vi "ziPollData.vi"(8 "Error In":errorcluster, 9 "Data In":T1, 10 "TimeOut ms (50)":i32=50, 11 "Handle In":T3 {"Handle" format="0x%08x"; "Conn" format="0x%08x"}) -> (0 "Error Out":errorcluster, 1 "Data Out":T1, 2 "PathArray":string[](array[string]), 3 "Handle Out":T3 {"Handle" format="0x%08x"; "Conn" format="0x%08x"}, 5 "Timed Out":bool, 7 "ziDataType":T4)   [LabVIEW 2015, in "Zurich Instruments LabOne.lvlib"]
doc: "This vi is <b>obsolete</b>. Use ziPollDataEx.vi in combination with ziGetEvent.vi instead.\n\nThis vi returns immediately if data is pending. Otherwise it waits for data for up to <b>TimeOut</b> milliseconds. All value changes that occur in nodes that have been subscribed to or in children of nodes that have been subscribed to, are sent from the Data Server to the ziAPI session. When no event was available within <b>TimeOut</b> milliseconds, the ziValueType field will be ZI_DATA_NONE and <b>Timed Out</b> will be true. Otherwise these fields hold the values corresponding to the event occurred."
uses:
  Zurich Instruments LabOne.lvlib
  Zurich Instruments/LabOne/API/LabVIEW/Zurich Instruments LabOne/Private/ziLV64.framework
  ziGetEventAuxInSample.vi
  ziGetEventDIOSample.vi
  ziGetEventScopeWave.vi
  ziGetEventByteArray.vi
  ziGetEventTreeChange.vi
  ziTypeDemodSample.ctl
  ziTypeHandle.ctl
  ziTypePollData.ctl
  ziTypePollType.ctl
panel:
  # "Obsolete (2013-11)\nUse ziPollDataEx instead"
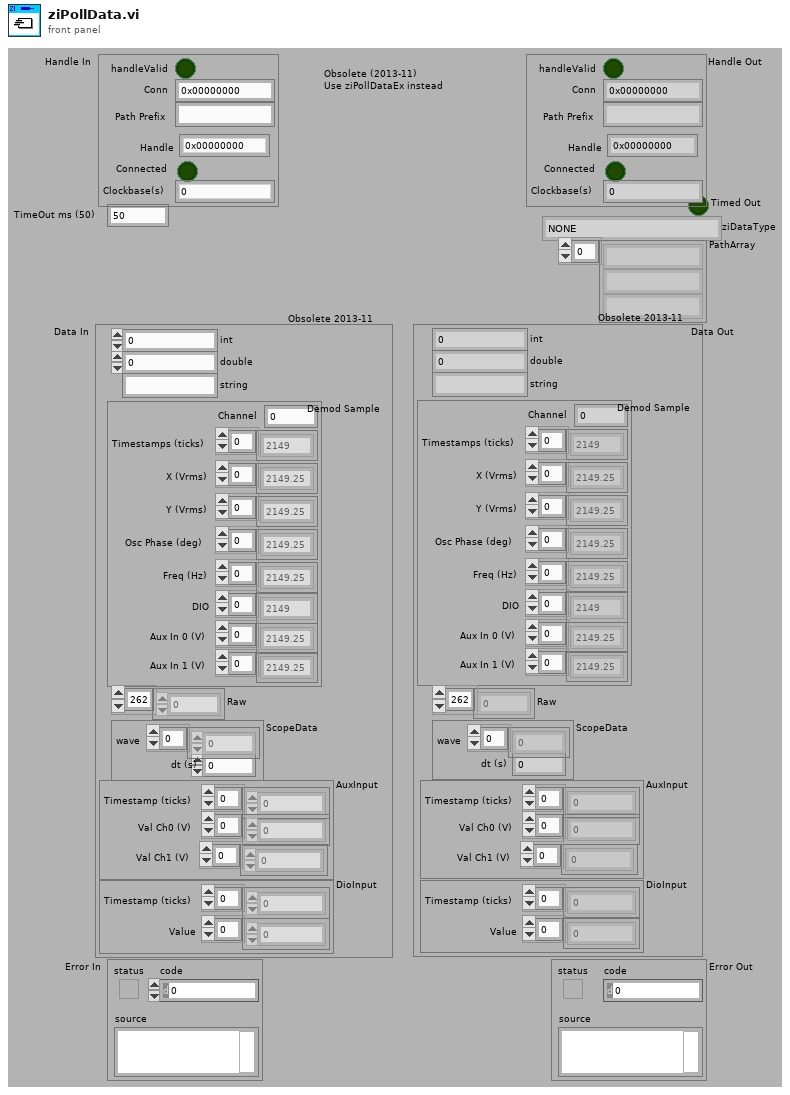
[diagram p1: front panel]
types:
  T1 = typedef "Zurich Instruments LabOne.lvlib/ziTypePollData.ctl" = cluster{"double":dbl, "Demod Sample":T2, "string":string, "Raw":u8[], "int":i32, "ScopeData":cluster{"wave":i16[], "dt (s)":dbl}, "DioInput":cluster{"Timestamp (ticks)":u64[], "Value":u32[]}, "AuxInput":cluster{"Timestamp (ticks)":u64[], "Val Ch0 (V)":dbl[], "Val Ch1 (V)":dbl[]}}
  T2 = typedef "Zurich Instruments LabOne.lvlib/ziTypeDemodSample.ctl" = cluster{"Channel":i32, "Timestamps (ticks)":u64[], "X (Vrms)":dbl[], "Y (Vrms)":dbl[], "Osc Phase (deg)":dbl[], "Freq (Hz)":dbl[], "DIO":u32[], "Aux In 0 (V)":dbl[], "Aux In 1 (V)":dbl[]}
  T3 = typedef "Zurich Instruments LabOne.lvlib/ziTypeHandle.ctl" = cluster{"handleValid":bool, "Conn":u64, "Path Prefix":string, "Handle":u64, "Connected":bool, "Clockbase(s)":dbl}
  T4 = typedef "Zurich Instruments LabOne.lvlib/ziTypePollType.ctl" = enum16{"NONE", "DOUBLE_DATA", "INTEGER_DATA", "DEMOD_SAMPLE", "SCOPE_WAVE_HF2", "AUXIN_SAMPLE", "DIO_SAMPLE", "BYTE_ARRAY", "PWA_WAVE", "9", "10", "11", "12", "13", "14", "15", "TREE_CHANGE_DEPRI", "17", "ERROR", "19", "20", "21", "22", "23", "24", "25", "26", "27", "28", "29", "30", "31", "DOUBLE_DATA_TS", "INTEGER_DATA_TS", "34", "SCOPE_WAVE", "36", "37", "BYTE_ARRAY_TS", "39", "40", "41", "42", "43", "44", "45", "CNT_DATA", "47", "TREE_CHANGE", "49", "50", "51", "52", "53", "54", "55", "56", "57", "58", "59", "60", "61", "62", "63", "SWEEPER_DATA", "SPECTRUM_DATA", "ADVISOR_DATA", "67", "IMP_DATA"}
  T5 = typedef "Zurich Instruments LabOne.lvlib/ziTypeScopeWave.ctl" = cluster{"Timestamp (ticks)":u64, "Timestamp Trigger (ticks)":u64, "dt (s)":dbl, "Channel Enable":u8[], "Channel Input":enum8{"Signal Input 1", "Signal Input 2", "Trigger Input 1", "Trigger Input 2", "Aux Output 1", "Aux Output 2", "Aux Output 3", "Aux Output 4", "Aux Input 1", "Aux Input 2"}[], "Trigger Enable":u64, "Trigger Input":u64, "Channel BW Limit":u8[], "Channel Math":u8[], "Channel Scaling":sgl[], "Sequence Number":u32, "Segment Number":u32, "Block Number":u32, "Data Transfer Mode":enum8{"Single Transfer", "Block Transfer", "Continuous Transfer", "FFT Single Transfer"}, "Block Marker":enum8{"None", "End of Block"}, "Flags":u8, "Sample Format":enum8{"Int16", "Int32", "Float32", "reserved", "Int16 Interleaved", "Int32 Interleaved", "Float32 Interleaved"}, "Sample Count":u32, "Channel Offset":dbl[], "Data Int16":i16[], "Data Int32":i32[], "Data Float":sgl[]}
  T6 = cluster{"Timestamp (ticks)":u64[], "Val Ch0 (V)":dbl[], "Val Ch1 (V)":dbl[]}
  T7 = typedef "Zurich Instruments LabOne.lvlib/ziTypeAuxInSample.ctl" = cluster{"Timestamp (ticks)":u64[], "Val Ch0 (V)":dbl[], "Val Ch1 (V)":dbl[]}
  T8 = cluster{"Timestamp (ticks)":u64[], "Value":u32[]}
  T9 = typedef "Zurich Instruments LabOne.lvlib/ziTypeByteArray.ctl" = cluster{"Timestamp (ticks)":u64, "bytes":i8[]}
  T10 = typedef "Zurich Instruments LabOne.lvlib/ziTypeTreeChange.ctl" = cluster{"Timestamp (ticks)":u64, "Action":enum32{"Remove", "Add", "Change"}, "Name":string}
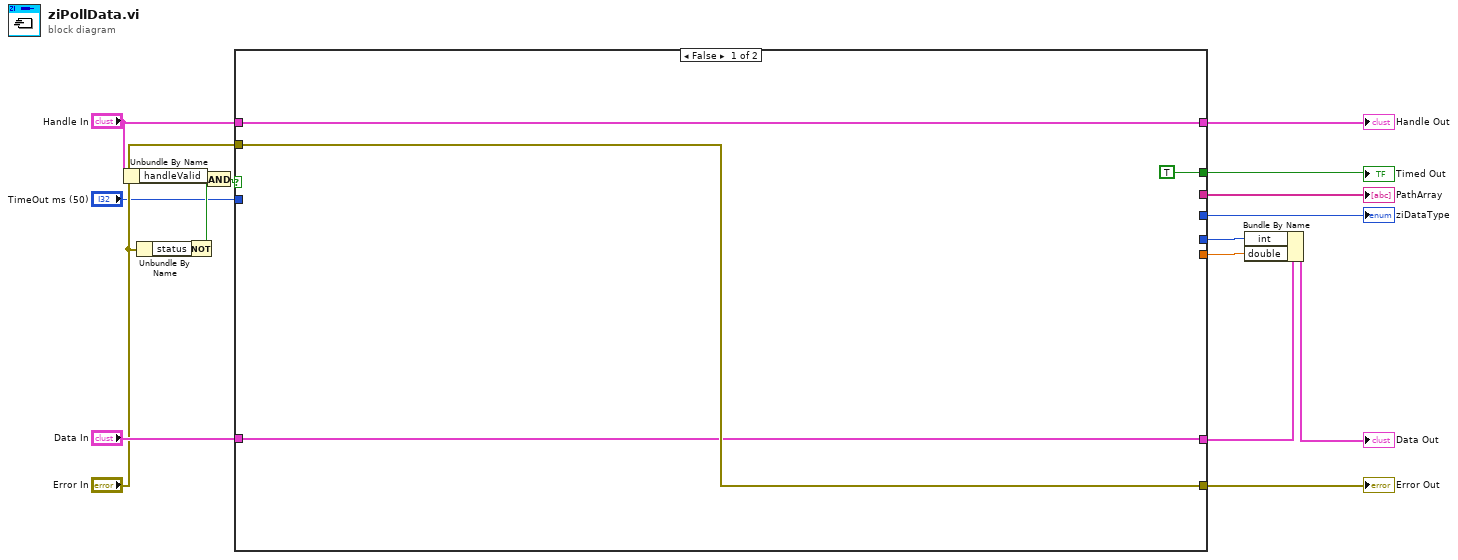
[diagram p0: block diagram]
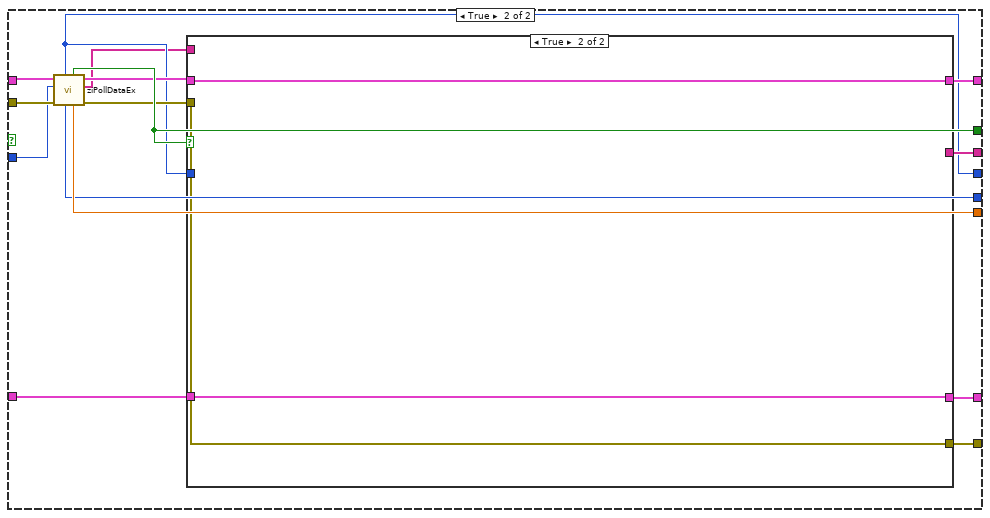
[diagram p2: hidden frame]
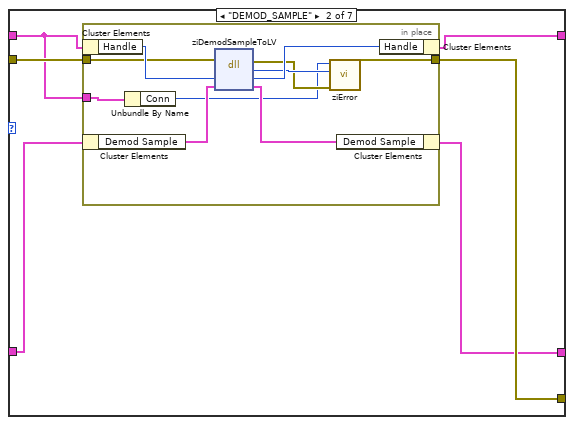
[diagram p4: hidden frame]
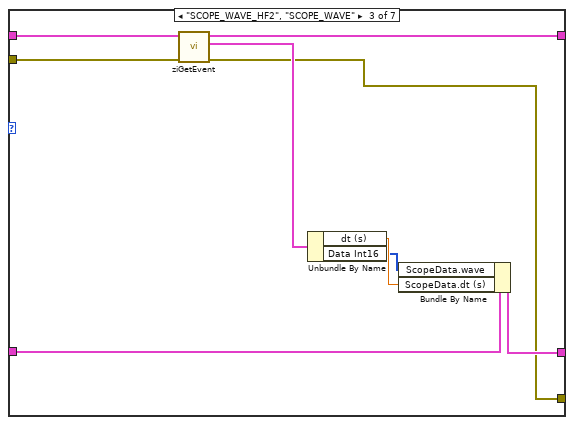
[diagram p5: hidden frame]
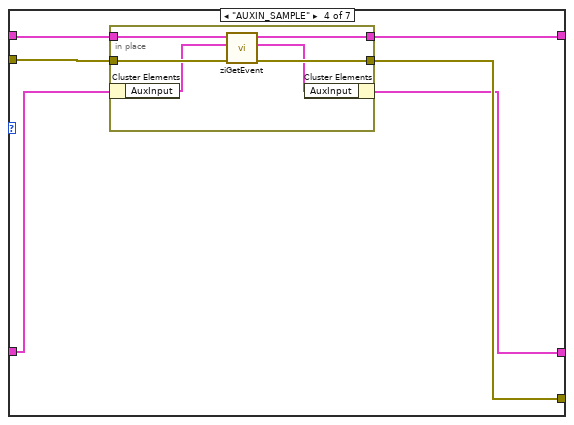
[diagram p6: hidden frame]
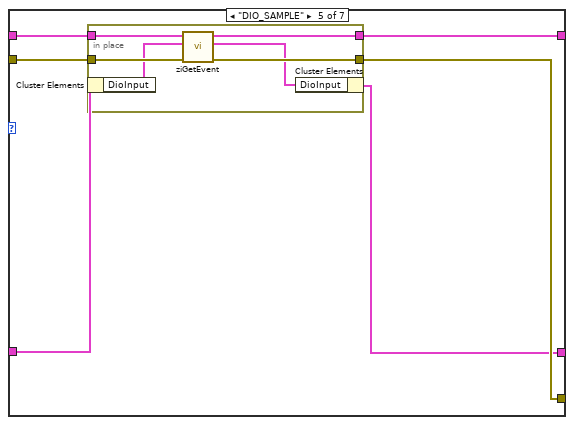
[diagram p7: hidden frame]
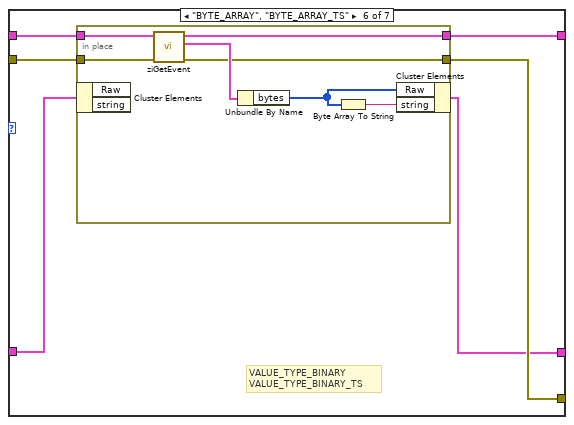
[diagram p8: hidden frame]
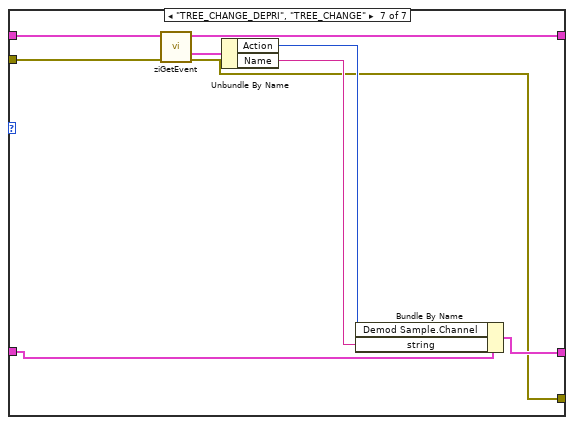
[diagram p9: hidden frame]
diagram:
  n1 = Unbundle By Name("Handle In") -> ("handleValid"=w10:bool)
  n2 = Unbundle By Name("Error In") -> ("status"=w9:bool)
  n3 = Not(x=w9) -> (.not. x?=w8:bool)
  n4 = And(x=w10, y=w8) -> (x .and. y?=w11:bool)
  n5 = case shown="False" w11 {
    tunnel: "Error In" -> [w21 w27]
    tunnel: [w21 w36] -> w17
    tunnel: [_ w35] -> w16
    tunnel: [TRUE w30] -> w12
    tunnel: "Data In" -> [w19 w34]
    tunnel: [w19 w33] -> w15
    tunnel: "Handle In" -> [w18 w31]
    tunnel: [w18 w32] -> w7
    tunnel: [_ w23] -> w6
    tunnel: [_ w24] -> w5
    tunnel: [_ w26] -> w4
    tunnel: "TimeOut ms (50)" -> [_ w25]
    frame False {
    }
    frame True {
      n6 = call "ziPollDataEx.vi"("error in"=w27, "Timeout ms (50)"=w25, "Handle In"=w31) -> ("error out"=w28:errorcluster, "PathArray"=w22:string[], "Handle Out"=w29:T3, "Value Double"=w26:dbl, "Timed Out"=w30:bool, "Value Int"=w24:i32, "ziValueType"=w23:T4)  [unwired: 1 in, 1 out]
      n7 = case shown="True" w30 {
        tunnel: w23 -> [w44 _]
        tunnel: w28 -> [w43 w121]
        tunnel: [w42 w121] -> w36
        tunnel: [w37 _] -> w35
        tunnel: w34 -> [w41 w120]
        tunnel: [w40 w120] -> w33
        tunnel: w29 -> [w39 w119]
        tunnel: [w38 w119] -> w32
        tunnel: w22 -> [w37 _]
        frame False {
          n8 = case shown="Default" w44 {
            tunnel: w43 -> [w47 w53 w70 w77 w89 w102 w112]
            tunnel: [w47 w52 w66 w75 w87 w99 w110] -> w42
            tunnel: w41 -> [w46 w51 w72 w74 w86 w98 w118]
            tunnel: [w46 w50 w71 w73 w85 w97 w117] -> w40
            tunnel: w39 -> [w45 w48 w65 w78 w90 w101 w116]
            tunnel: [w45 w49 w64 w76 w88 w100 w111] -> w38
            frame Default {
            }
            frame "DEMOD_SAMPLE" {
              n9 = in-place {
                in-place-border: w53 -> [w59]
                in-place-border: [w57] -> w52
                in-place-border: w48 -> [w55]
                n10 = in-place-cluster #1(w48) -> ("Handle"=w62:u64)
                n11 = in-place-cluster #2(w51) -> ("Demod Sample"=w63:T2)
                n12 = Unbundle By Name(w55) -> ("Conn"=w54:u64)
                n13 = dll-call lib="Users/arkady/Desktop/ado/github/resonant_ultrasound_arxiv/maglab ultrasound -- arkady --arxiv/Zurich Instruments/LabOne/API/LabVIEW/Zurich Instruments LabOne/Private/ziLV*.*" fn="ziDemodSampleToLV"(error in=w59, "ziEventBuffer"=w62, "DemodSample"=w63) -> (error out=w58:errorcluster, "return type"=w60:u32, "ziEventBuffer"=w61:u64, "DemodSample"=w56:T2)  [unwired: 2 in, 1 out]
                n14 = call "ziError.vi"("Conn"=w54, "ziErrorCode"=w60, "Error In"=w58) -> ("Error Out"=w57:errorcluster)  [unwired: 2 in, 1 out]
                n15 = in-place-cluster #2("Demod Sample"=w56) -> (w50:T1)
                n16 = in-place-cluster #1("Handle"=w61) -> (w49:T3)
              }
            }
            frame "SCOPE_WAVE_HF2", "SCOPE_WAVE" {
              n17 = call-poly "ziGetEvent.vi"("Error In"=w70, "Handle In"=w65) -> ("Error Out"=w66:errorcluster, "ScopeWave Out"=w69:T5, "Handle Out"=w64:T3)  [unwired: 7 in]
              n18 = Unbundle By Name(w69) -> ("dt (s)"=w68:dbl, "Data Int16"=w67:i16[])
              n19 = Bundle By Name(cluster=w72, "ScopeData.wave"=w67, "ScopeData.dt (s)"=w68) -> (w71:T1)
            }
            frame "AUXIN_SAMPLE" {
              n20 = in-place {
                in-place-border: w78 -> [w84]
                in-place-border: w77 -> [w83]
                in-place-border: [w82] -> w76
                in-place-border: [w81] -> w75
                n21 = in-place-cluster #3(w74) -> ("AuxInput"=w80:T6)
                n22 = call-poly "ziGetEvent.vi"("Error In"=w83, "AuxIn In"=w80, "Handle In"=w84) -> ("Error Out"=w81:errorcluster, "AuxIn Out"=w79:T7, "Handle Out"=w82:T3)  [unwired: 6 in]
                n23 = in-place-cluster #3("AuxInput"=w79) -> (w73:T1)
              }
            }
            frame "DIO_SAMPLE" {
              n24 = in-place {
                in-place-border: w90 -> [w96]
                in-place-border: w89 -> [w95]
                in-place-border: [w94] -> w88
                in-place-border: [w93] -> w87
                n25 = in-place-cluster #4(w86) -> ("DioInput"=w92:T8)
                n26 = call-poly "ziGetEvent.vi"("Error In"=w95, "DIOIn"=w92, "Handle In"=w96) -> ("Error Out"=w93:errorcluster, "DIO Out"=w91:T8, "Handle Out"=w94:T3)  [unwired: 6 in]
                n27 = in-place-cluster #4("DioInput"=w91) -> (w85:T1)
              }
            }
            frame "BYTE_ARRAY", "BYTE_ARRAY_TS" {
              # "VALUE_TYPE_BINARY\nVALUE_TYPE_BINARY_TS"
              n28 = in-place {
                in-place-border: w102 -> [w109]
                in-place-border: w101 -> [w108]
                in-place-border: [w107] -> w100
                in-place-border: [w105] -> w99
                n29 = in-place-cluster #5(w98) -> ()  [unwired: 2 out]
                n30 = call-poly "ziGetEvent.vi"("Error In"=w109, "Handle In"=w108) -> ("Error Out"=w105:errorcluster, "ByteArray Out"=w106:T9, "Handle Out"=w107:T3)  [unwired: 7 in]
                n31 = Unbundle By Name(w106) -> ("bytes"=w104:i8[])
                n32 = Byte Array To String(unsigned byte array=w104) -> (string=w103:string)
                n33 = in-place-cluster #5("Raw"=w104, "string"=w103) -> (w97:T1)
              }
            }
            frame "TREE_CHANGE_DEPRI", "TREE_CHANGE" {
              n34 = call-poly "ziGetEvent.vi"("Error In"=w112, "Handle In"=w116) -> ("Error Out"=w110:errorcluster, "TreeChange Out"=w115:T10, "Handle Out"=w111:T3)  [unwired: 7 in]
              n35 = Unbundle By Name(w115) -> ("Action"=w113:enum32{"Remove", "Add", "Change"}, "Name"=w114:string)
              n36 = Bundle By Name(cluster=w118, "Demod Sample.Channel"=w113, "string"=w114) -> (w117:T1)
            }
          }
        }
        frame True {
        }
      }
    }
  }
  "Error Out" <- w17
  "ziDataType" <- w6
  "Timed Out" <- w12
  "Handle Out" <- w7
  "PathArray" <- w16
  n37 = Bundle By Name(cluster=w15, "int"=w5, "double"=w4) -> (→"Data Out":T1)
